vi "Initialize.vi"(8 "error in":errorcluster, 11 "Physical channels in":string="PCI-1751,BID#0/port0:5") -> (0 "error out":errorcluster, 3 "task out":i32)   [LabVIEW 2025, in "DO_Relay.lvlib"]
uses:
  DO_Relay.lvlib
  <userlib>/DAQNavi Polymorphic VI/create/DAQNavi Create Channel(DO-Digital Output).vi
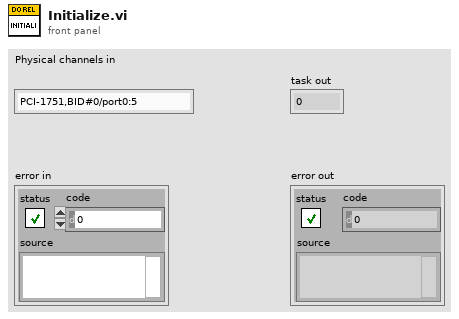
[diagram p1: front panel]
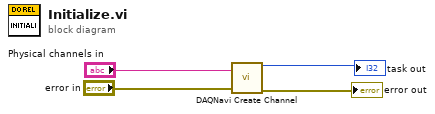
[diagram p0: block diagram]
diagram:
  n1 = call-poly <userlib>:"DAQNavi Create Channel.vi"("physical channels"="Physical channels in", "error in (no error)"="error in") -> ("task out"=→"task out":i32, "error out"=→"error out":errorcluster)  [unwired: 3 in, 9 out]
